vi "Mind Reading Core.vi"(10 "FirstRun":bool, 11 "Answer":T1) -> (1 "Results generated":bool, 2 "Possible Results":string[](array[string]), 3 "AI Question":string)   [LabVIEW 2015]
uses:
  Data Def/Answer.ctl
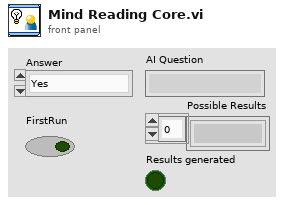
[diagram p1: front panel]
types:
  T1 = typedef "Answer.ctl" = enum16{"Yes", "No", "I don't Know"}
  T2 = typedef "Classify.ctl" = cluster{"Item":string, "Count":i32, "Athletics":string[]}
  T3 = typedef "Question Index.ctl" = cluster{"row":i32, "col":i32}
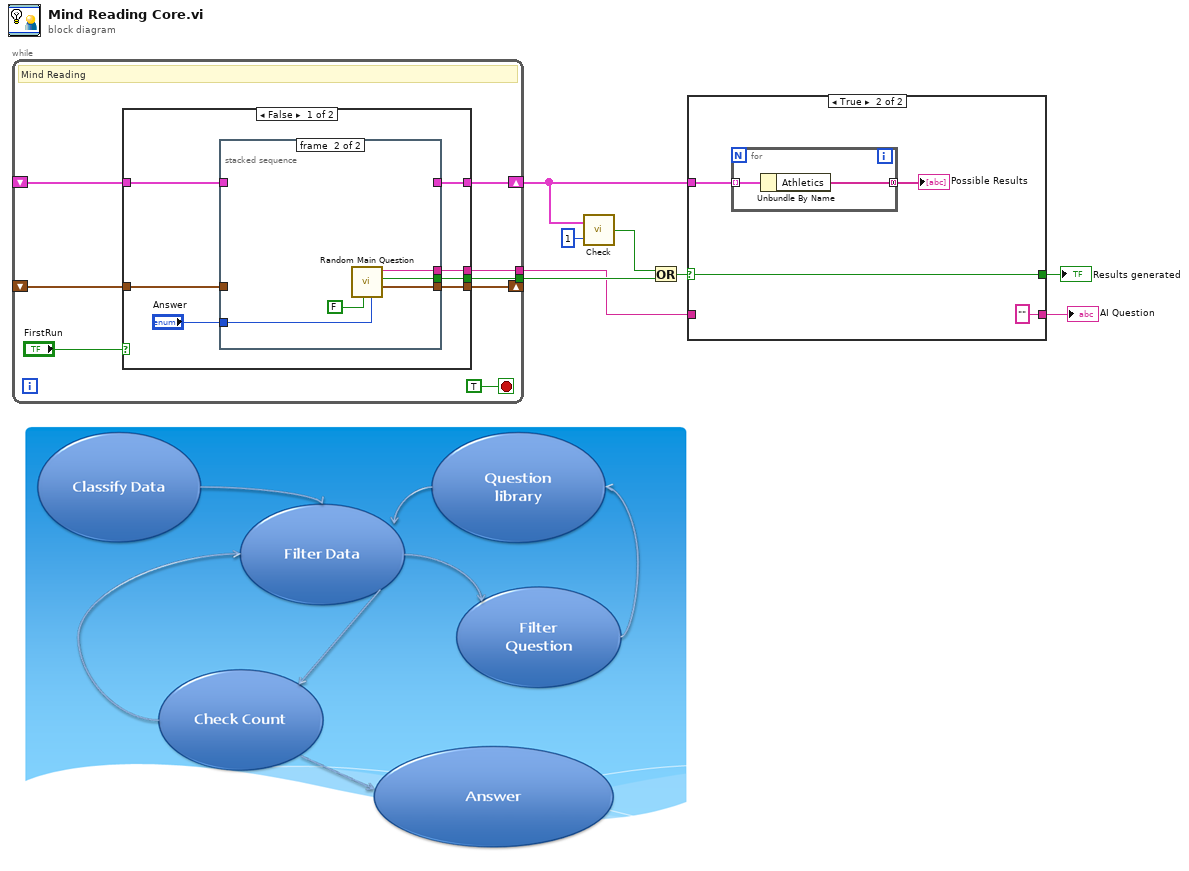
[diagram p0: block diagram]
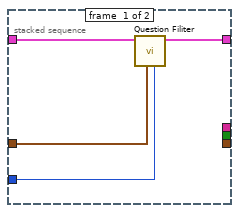
[diagram p3: hidden frame]
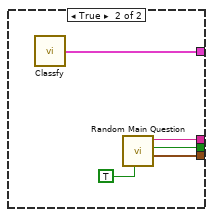
[diagram p4: hidden frame]
diagram:
  n1 = while {
    shift-right: [w14] -> w8
    shift-left: _ -> [w13]
    tunnel: [w12] -> w3
    tunnel: [w11] -> w2
    shift-right: [w10] -> _
    shift-left: _ -> [w9]
    stop <- TRUE stop-if-true
    # "Mind Reading"
    n2 = case shown="False" "FirstRun" {
      tunnel: [w23 w37] -> w14
      tunnel: w13 -> [w22 _]
      tunnel: [w20 w36] -> w11
      tunnel: [w19 w35] -> w12
      tunnel: [w18 w33] -> w10
      tunnel: w9 -> [w17 _]
      frame False {
        n3 = stacked-sequence {
          tunnel: [w27 _] -> w23
          tunnel: w22 -> [w26 _]
          tunnel: "Answer" -> [w25 w32]
          tunnel: [_ w30] -> w20
          tunnel: [_ w29] -> w19
          tunnel: [_ w28] -> w18
          tunnel: w17 -> [w24 _]
          frame #0 {
            n4 = call "Question Filiter.vi"("Answer"=w25, "Question Index"=w24, "Classfy In"=w26) -> ("Classfy Out"=w27:T2[])  [unwired: 8 in]
          }
          frame #1 {
            n5 = call "Random Main Question.vi"("Answer"=w32, "Fist Run?"=FALSE) -> ("Question Index"=w28:T3, "End"=w29:bool, "AI Question"=w30:string)  [unwired: 7 in]
          }
        }
      }
      frame True {
        n6 = call "Classfy.vi"() -> ("Classfy 1"=w37:T2[])  [unwired: 1 in]
        n7 = call "Random Main Question.vi"("Fist Run?"=TRUE) -> ("Question Index"=w33:T3, "End"=w35:bool, "AI Question"=w36:string)  [unwired: 8 in]
      }
    }
  }
  n8 = call "Check.vi"("Limit"=1, "Classfy"=w8) -> ("End"=w7:bool)
  n9 = Or(x=w7, y=w3) -> (x .or. y?=w6:bool)
  n10 = case shown="True" w6 {
    selector: w6 -> [w39 w41]
    tunnel: w8 -> [_ w43]
    tunnel: [w39 w41] -> w5
    tunnel: w2 -> [w38 _]
    tunnel: [w38 "" ("AI Question")] -> w1
    frame False {
    }
    frame True {
      n11 = for {
        tunnel: w43 -> [w45] mode=indexing
        tunnel: [w44] -> w42 mode=concatenating
        n12 = Unbundle By Name(w45) -> ("Athletics"=w44:string[])
      }
      "Possible Results" <- w42
    }
  }
  "Results generated" <- w5
  "AI Question" <- w1
